vi "Average Measure (DT).vi"(0 "VISA resource name":refnum<visa-resource-name>, 5 "Channel1 (1: Channel 1)":u16(ring)=1 items=["Channel 1"=1, "Channel 2"=2, "Channel 3"=3, "Channel 4"=4, "Function 1"=5, "Function 2"=6, "Function 3"=7, "Function 4"=8, "Memory 1"=9, "Memory 2"=10, "Memory 3"=11, "Memory 4"=12], 7 "Channel2 (2: Channel 2)":u16(ring)=2 items=["Channel 1"=1, "Channel 2"=2, "Channel 3"=3, "Channel 4"=4, "Function 1"=5, "Function 2"=6, "Function 3"=7, "Function 4"=8, "Memory 1"=9, "Memory 2"=10, "Memory 3"=11, "Memory 4"=12], 9 "Maximum Time (10000ms)":u32=10000, 11 "error in (no error)":errorcluster, 12 "Averages":u32=32, 13 "Max Errors":u32=40) -> (4 "VISA resource name out":refnum<visa-resource-name>, 6 "Measure Average":dbl caption="Measurement", 8 "Measure Error":dbl caption="Measurement", 15 "error out":errorcluster)   [LabVIEW 2009]
uses:
  <instrlib>/Agilent 8000 Series/Public/Data/Read Measurement (Delta Time).vi
  <instrlib>/Agilent 8000 Series/Agilent 8000 Series.lvlib
  <vilib>/Analysis/NI_AALBase.lvlib
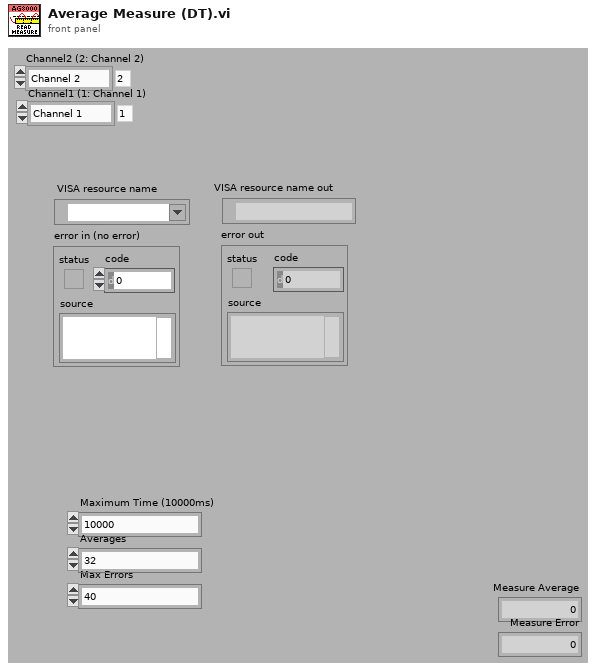
[diagram p1: front panel]
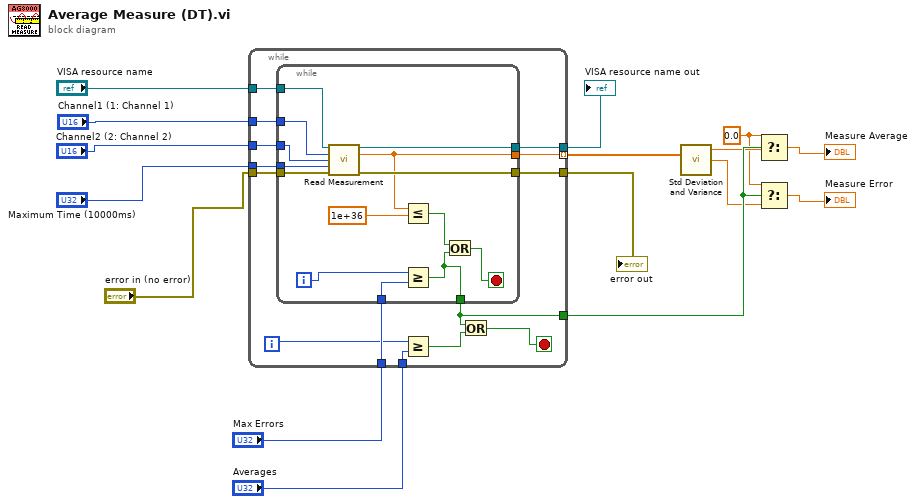
[diagram p0: block diagram]
diagram:
  w5 = 0.0 ("t")
  n1 = while {
    tunnel: "VISA resource name" -> [w30]
    tunnel: "Maximum Time (10000ms)" -> [w29]
    tunnel: "error in (no error)" -> [w28]
    tunnel: [w27] -> w13
    tunnel: [w26] -> w9 mode=indexing
    tunnel: [w25] -> w12
    tunnel: "Max Errors" -> [w24]
    tunnel: "Averages" -> [w22]
    tunnel: [w19] -> w8
    tunnel: "Channel2 (2: Channel 2)" -> [w18]
    tunnel: "Channel1 (1: Channel 1)" -> [w17]
    i -> [w23]
    stop <- w20 stop-if-true
    n2 = while {
      tunnel: w30 -> [w44]
      tunnel: w29 -> [w43]
      tunnel: w28 -> [w42]
      tunnel: [w41] -> w27
      tunnel: [w39] -> w26
      tunnel: [w40] -> w25
      tunnel: w24 -> [w35]
      tunnel: [w33] -> w19
      tunnel: w18 -> [w32]
      tunnel: w17 -> [w31]
      i -> [w36]
      stop <- w34 stop-if-true
      n3 = call-poly <instrlib>:"Read Measurement.vi"("VISA resource name"=w44, "Channel1 (1: Channel 1)"=w31, "Channel2 (2: Channel 2)"=w32, "Maximum Time (10000ms)"=w43, "error in (no error)"=w42) -> ("VISA resource name out"=w40:refnum<visa-resource-name>, "Delta Time(s)"=w39:dbl, "error out"=w41:errorcluster)  [unwired: 8 in]
      n4 = Less Or Equal?(x=w39, y=1e+36) -> (x <= y?=w38:bool)
      n5 = Greater Or Equal?(x=w36, y=w35) -> (x >= y?=w33:bool)
      n6 = Or(x=w38, y=w33) -> (x .or. y?=w34:bool)
    }
    n7 = Greater Or Equal?(x=w23, y=w22) -> (x >= y?=w21:bool)
    n8 = Or(x=w19, y=w21) -> (x .or. y?=w20:bool)
  }
  "error out" <- w13
  "VISA resource name out" <- w12
  n9 = call <vilib>:"Std Deviation and Variance.vi"("X"=w9) -> ("mean"=w6:dbl, "standard deviation"=w7:dbl)  [unwired: 1 in, 1 out]
  n10 = Select(t=w5, s=w8, f=w6) -> (s? t:f=→"Measure Average":dbl)
  n11 = Select(t=w5, s=w8, f=w7) -> (s? t:f=→"Measure Error":dbl)
